vi "MTS_U32ToRGB.vi"(10 "Color":u32) -> (1 "Blue":u8, 2 "Green":u8, 3 "Red":u8)   [LabVIEW 2011]
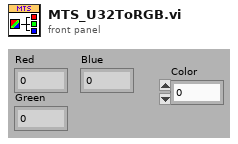
[diagram p1: front panel]
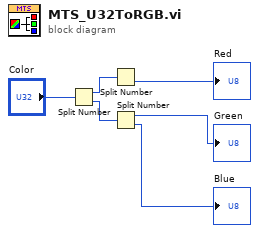
[diagram p0: block diagram]
diagram:
  n1 = Split Number(x="Color") -> (hi(x)=w5:u16, lo(x)=w4:u16)
  n2 = Split Number(x=w5) -> (lo(x)=→"Red":u8)  [unwired: 1 out]
  n3 = Split Number(x=w4) -> (hi(x)=→"Green":u8, lo(x)=→"Blue":u8)
